vi "Label.vi"(8 "error in (no error)":errorcluster, 10 "Label":T1, 11 "ITX Commands in":refnum<class "ITX Commands.lvclass">) -> (0 "error out":errorcluster, 3 "ITX Commands out":refnum<class "ITX Commands.lvclass">)   [LabVIEW 2019, in "ITX Commands.lvclass"]
uses:
  ITX Commands.lvclass
  typedefs/Label--cluster.ctl
panel:
  out "resulting string":string
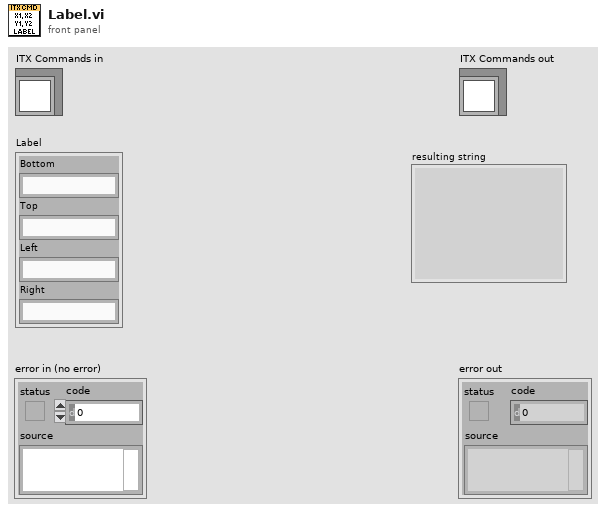
[diagram p1: front panel]
types:
  T1 = typedef "ITX Commands.lvclass/Label--cluster.ctl" = cluster{"Bottom":string, "Top":string, "Left":string, "Right":string}
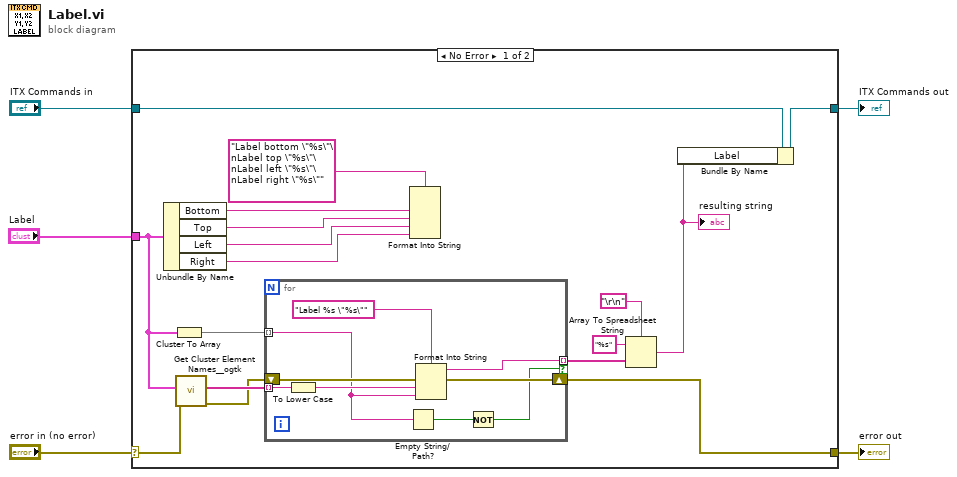
[diagram p0: block diagram]
diagram:
  n1 = case shown="No Error" "error in (no error)" {
    selector: "error in (no error)" -> [w15 w33]
    tunnel: [w10 w33] -> w4
    tunnel: [w16 w32] -> w2
    tunnel: "ITX Commands in" -> [w22 w32]
    tunnel: "Label" -> [w14 _]
    frame No Error {
      n2 = Unbundle By Name(w14) -> ("Bottom"=w20:string, "Top"=w19:string, "Left"=w18:string, "Right"=w17:string)
      n3 = Cluster To Array(cluster=w14) -> (array=w13:string[])
      n4 = call "Get Cluster Element Names__ogtk.vi"("error in (no error)"=w15, "Cluster"=w14) -> ("error out"=w11:errorcluster, "Element Names"=w12:string[])  [unwired: 8 in]
      n5 = for {
        tunnel: w13 -> [w25] mode=indexing
        tunnel: w12 -> [w30] mode=indexing
        shift-right: [w27] -> w10
        shift-left: w11 -> [w28]
        tunnel: [w26] -> w9 mode=indexing if=w23
        n6 = To Lower Case(string=w30) -> (all lower case string=w29:string)
        n7 = Empty String/Path?(string/path=w25) -> (empty?=w24:bool)
        n8 = Format Into String(format string="Label %s \"%s\"", error in=w28, w29, w25) -> (resulting string=w26:string, error out=w27:errorcluster)  [unwired: 1 in]
        n9 = Not(x=w24) -> (.not. x?=w23:bool)
      }
      n10 = Format Into String(format string="Label bottom \"%s\"\nLabel top \"%s\"\nLabel left \"%s\"\nLabel right \"%s\"", w20, w19, w18, w17) -> ()  [unwired: 2 in, 2 out]
      n11 = Array To Spreadsheet String(delimiter (Tab)="\r\n", array=w9, 3:"%s" ("format string")) -> (spreadsheet string=w7:string)
      "resulting string" <- w7
      n12 = Bundle By Name(cluster=w22, "Label"=w7) -> (w16:refnum<class "ITX Commands.lvclass">)
    }
    frame Error {
    }
  }
  "error out" <- w4
  "ITX Commands out" <- w2
